vi "Set value by string.vi"(8 "error in (no error)":errorcluster, 10 "Value":string, 11 "Column in":refnum<class "By-Value Column.lvclass">) -> (0 "error out":errorcluster, 3 "Column out":refnum<class "By-Value Column.lvclass">)   [LabVIEW 2020, in "Basic Columns.lvlib" / "By-Value Column.lvclass"]
uses:
  By-Value Column.lvclass
  By-Value Column.lvclass/By-Value Column.ctl
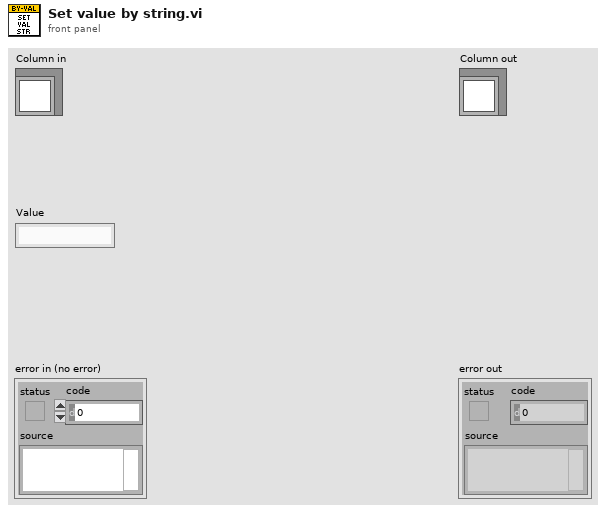
[diagram p1: front panel]
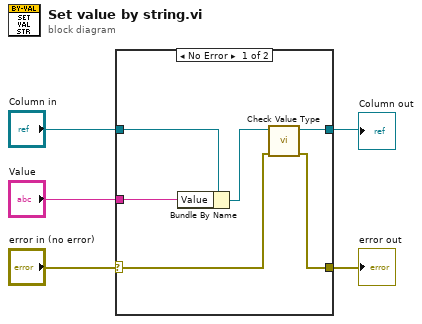
[diagram p0: block diagram]
diagram:
  n1 = case shown="No Error" "error in (no error)" {
    selector: "error in (no error)" -> [w7 w12]
    tunnel: [w6 w12] -> w1
    tunnel: "Column in" -> [w11 w13]
    tunnel: [w8 w13] -> w5
    tunnel: "Value" -> [w10 _]
    frame No Error {
      n2 = Bundle By Name(cluster=w11, "Value"=w10) -> (w9:refnum<class "By-Value Column.lvclass">)
      n3 = call-dynamic "Check Value Type.vi"("error in (no error)"=w7, "Column in"=w9) -> ("error out"=w6:errorcluster, "Column out"=w8:refnum<class "By-Value Column.lvclass">)  [unwired: 8 in]
    }
    frame Error {
    }
  }
  "error out" <- w1
  "Column out" <- w5
